vi "Position_Three_Scoring.vi"(11 "data string":string) -> (3 "String":string)   [LabVIEW 2012, in "Serenity_mk2.lvrbt"]
uses:
  Serenity_mk2.lvrbt
  State_Typ.ctl
  auto_drive_TYP.ctl
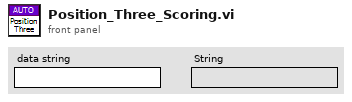
[diagram p1: front panel]
types:
  T1 = typedef "auto_drive_TYP.ctl" = cluster{"Left X":i8, "Left Y":i8, "Right Y":i8, "Power (100)":i8, "Wait (ms)":u32, "Enc/Deg Target":i32, "Move Type":enum16{"Relative Degrees", "Wait", "Encoder"}}
  T2 = typedef "State_Typ.ctl" = enum16{"Stop", "Check for Position 3", "Check for Position 2", "Move", "Reset Enc", "Read Enc", "Lift", "Dump Close"}
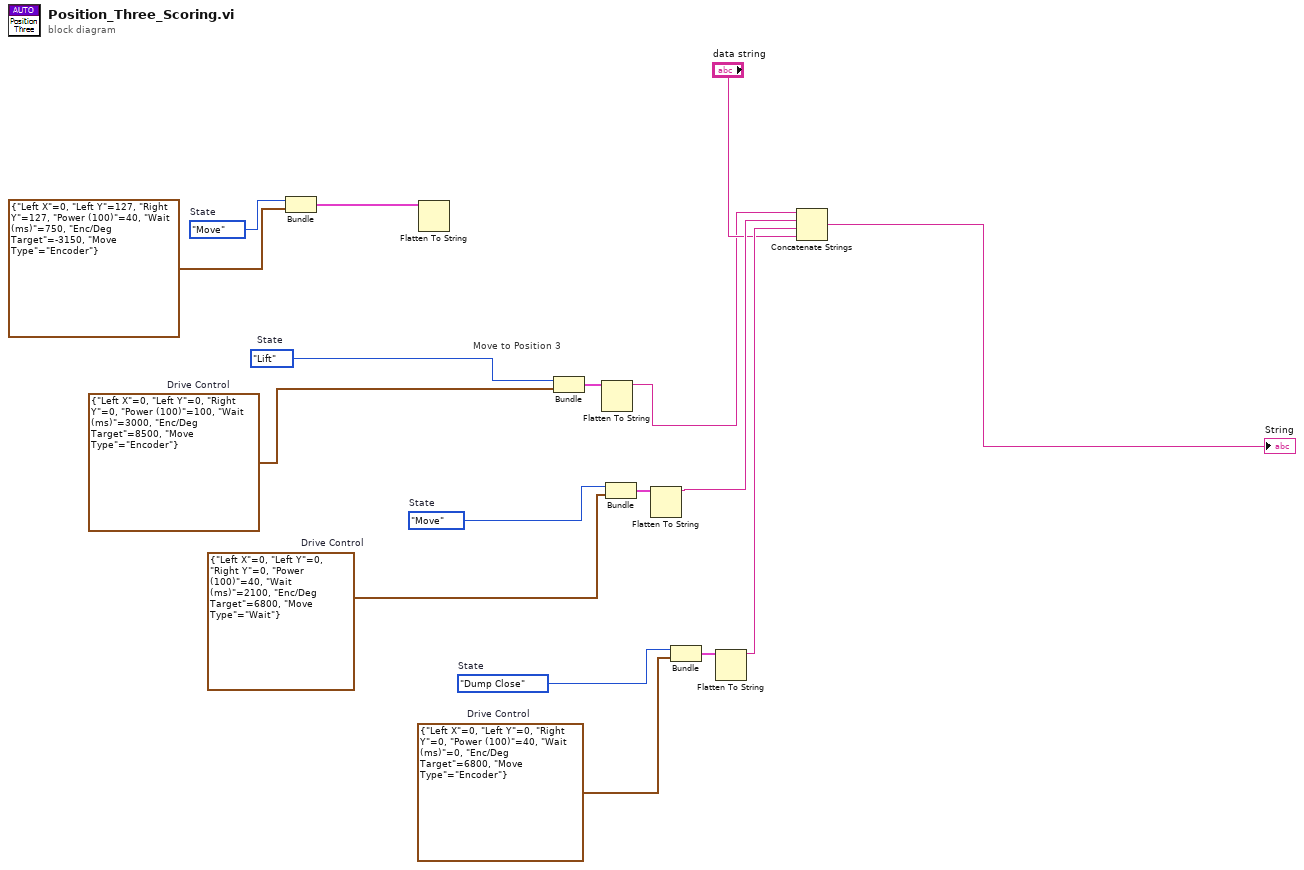
[diagram p0: block diagram]
diagram:
  w15 = T1 {"Left X"=0, "Left Y"=0, "Right Y"=0, "Power (100)"=40, "Wait (ms)"=2100, "Enc/Deg Target"=6800, "Move Type"=enum."Wait"}  # Drive Control
  w14 = State_Typ."Move"  # State
  w10 = State_Typ."Move"  # State
  w9 = T1 {"Left X"=0, "Left Y"=0, "Right Y"=0, "Power (100)"=100, "Wait (ms)"=3000, "Enc/Deg Target"=8500, "Move Type"=enum."Encoder"}  # Drive Control
  w3 = T1 {"Left X"=0, "Left Y"=0, "Right Y"=0, "Power (100)"=40, "Wait (ms)"=0, "Enc/Deg Target"=6800, "Move Type"=enum."Encoder"}  # Drive Control
  w2 = State_Typ."Dump Close"  # State
  w1 = State_Typ."Lift"  # State
  # "Move to Position 3"
  n1 = Bundle("State"=w10, "Drive Control"=T1 {"Left X"=0, "Left Y"=127, "Right Y"=127, "Power (100)"=40, "Wait (ms)"=750, "Enc/Deg Target"=-3150, "Move Type"=enum."Encoder"}) -> (w11:cluster{"State":T2, "Drive Control":T1})  [unwired: 1 in]
  n2 = Flatten To String(anything=w11) -> ()  [unwired: 3 in, 3 out]
  n3 = Bundle("State"=w1, "Drive Control"=w9) -> (w4:cluster{"State":T2, "Drive Control":T1})  [unwired: 1 in]
  n4 = Flatten To String(anything=w4) -> (data string=w6:string)  [unwired: 3 in, 2 out]
  n5 = Bundle("State"=w14, "Drive Control"=w15) -> (w16:cluster{"State":T2, "Drive Control":T1})  [unwired: 1 in]
  n6 = Flatten To String(anything=w16) -> (data string=w17:string)  [unwired: 3 in, 2 out]
  n7 = Bundle("State"=w2, "Drive Control"=w3) -> (w5:cluster{"State":T2, "Drive Control":T1})  [unwired: 1 in]
  n8 = Flatten To String(anything=w5) -> (data string=w13:string)  [unwired: 3 in, 2 out]
  n9 = Concatenate Strings(w6, w17, w13, "data string") -> (→"String":string)
